vi "Final Cleanup.vi"(8 "error in (no error)":errorcluster, 9 "initial selection list in":refnum<vi>[](array[refnum]), 10 "case structure in":refnum<vi>, 11 "VI in":refnum<vi>) -> (0 "error out":errorcluster, 1 "initial selection list out":refnum<vi>[](array[refnum]), 2 "case structure out":refnum<vi>, 3 "VI out":refnum<vi>)   [LabVIEW 2017]
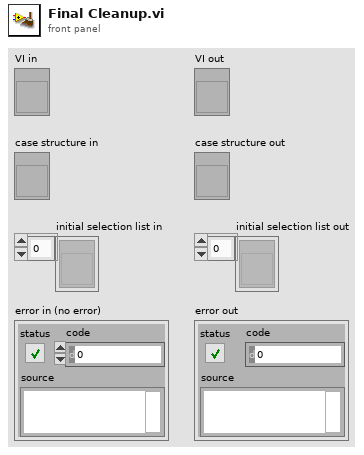
[diagram p1: front panel]
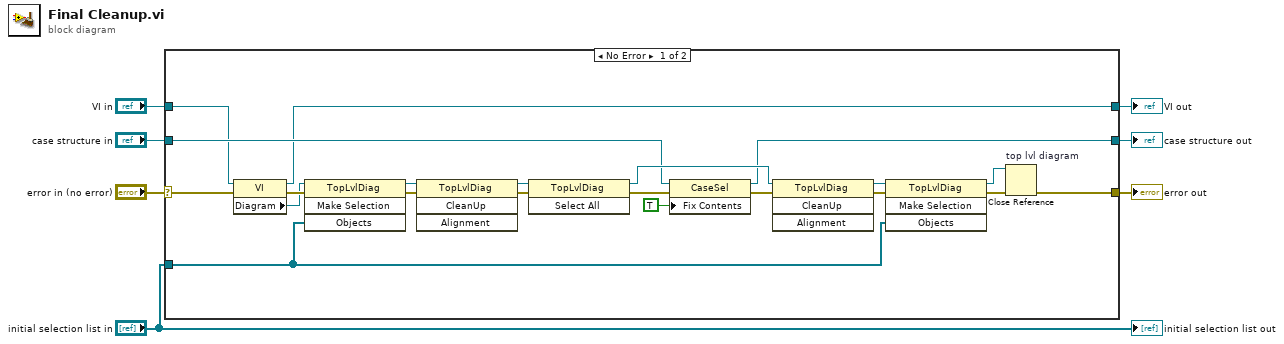
[diagram p0: block diagram]
diagram:
  n1 = case shown="No Error" "error in (no error)" {
    selector: "error in (no error)" -> [w8 w31]
    tunnel: "case structure in" -> [w19 w29]
    tunnel: [w16 w29] -> w6
    tunnel: "initial selection list in" -> [w14 _]
    tunnel: "VI in" -> [w12 w30]
    tunnel: [w11 w30] -> w3
    tunnel: [w10 w31] -> w2
    frame No Error {
      n2 = property class="VI"(reference=w12, error in=w8) -> (reference out=w11:refnum<vi>, error out=w28:errorcluster, "Diagram"=w13:refnum<vi>)
      n3 = invoke class="TopLvlDiag" method="Make Selection"(reference=w13, error in=w28, "Objects"=w14) -> (reference out=w17:refnum<vi>, error out=w18:errorcluster)  [unwired: 1 in, 2 out]
      n4 = invoke class="TopLvlDiag" method="CleanUp"(reference=w17, error in=w18) -> (reference out=w24:refnum<vi>, error out=w21:errorcluster)  [unwired: 2 in, 2 out]
      n5 = invoke class="TopLvlDiag" method="Select All"(reference=w24, error in=w21) -> (reference out=w25:refnum<vi>, error out=w23:errorcluster)  [unwired: 1 in, 1 out]
      n6 = property class="CaseSel"(reference=w19, error in=w23, "Fix Contents"=TRUE) -> (reference out=w16:refnum<vi>, error out=w22:errorcluster)
      n7 = invoke class="TopLvlDiag" method="CleanUp"(reference=w25, error in=w22) -> (reference out=w26:refnum<vi>, error out=w27:errorcluster)  [unwired: 2 in, 2 out]
      n8 = invoke class="TopLvlDiag" method="Make Selection"(reference=w26, error in=w27, "Objects"=w14) -> (reference out=w9:refnum<vi>, error out=w15:errorcluster)  [unwired: 1 in, 2 out]
      n9 = Close Reference "top lvl diagram"(reference=w9, error in (no error)=w15) -> (error out=w10:errorcluster)
    }
    frame Error {
    }
  }
  "case structure out" <- w6
  "error out" <- w2
  "VI out" <- w3
  "initial selection list out" <- "initial selection list in"
